vi "Timer_Restart.vi"(8 "Pass_Through_Time":dbl=-1.0 format="%33.4f", 11 "in Timer":T1 {"Accumulated TIme" format="%13.5p"; "StartTime" format="%13.5p"}) -> (3 "out Timer":T1 {"Accumulated TIme" format="%13.5p"; "StartTime" format="%13.5p"})   [LabVIEW 2019, in "Trajectory_Library.lvlib"]
doc: "Restart the timer by stopping the timer, if it is not already stopped, resetting the accumulated time, then starting the timer again. If you want an event to periodically reoccur at some time interval from the start time, consider using HasPeriodPassed instead.\n\nInputs:\n - Timer -- The Timer data cluster\n\nOutputs:\n - Timer -- The modified Timer data cluster"
uses:
  Trajectory_Library.lvlib
  TypeDef/TIMER.ctl
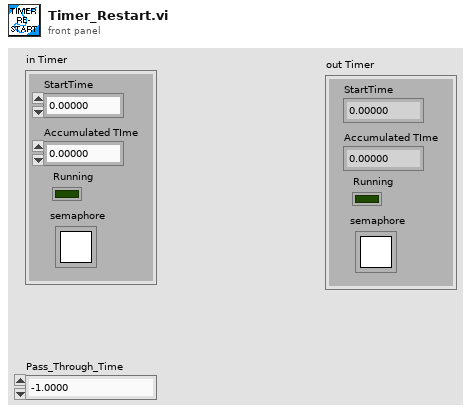
[diagram p1: front panel]
types:
  T1 = typedef "Trajectory_Library.lvlib/TIMER.ctl" = cluster{"StartTime":dbl, "Accumulated TIme":dbl, "Running":bool, "semaphore":T2}
  T2 = typedef "Semaphore RefNum" = refnum<k1>
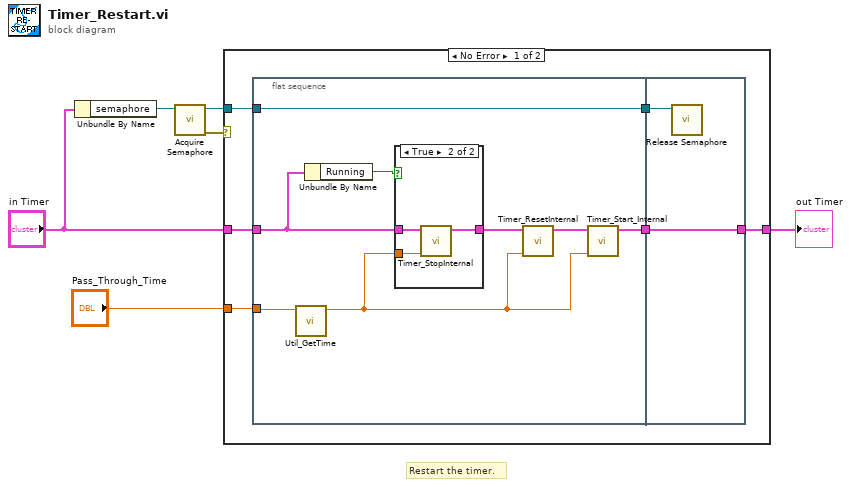
[diagram p0: block diagram]
diagram:
  # "Restart the timer."
  n1 = Unbundle By Name("in Timer") -> ("semaphore"=w4:T2)
  n2 = call <vilib>:"Acquire Semaphore.vi"("semaphore"=w4) -> ("error out"=w3:errorcluster, "semaphore out"=w2:T2)  [unwired: 4 in, 1 out]
  n3 = case shown="No Error" w3 {
    tunnel: "in Timer" -> [w12 w27]
    tunnel: [w11 w27] -> w6
    tunnel: w2 -> [w8 _]
    tunnel: "Pass_Through_Time" -> [w7 _]
    frame No Error {
      n4 = flat-sequence {
        tunnel: w12 -> [w17]
        tunnel: [w14] -> w10
        tunnel: [w20] -> w9
        tunnel: w8 -> [w20]
        tunnel: w7 -> [w16]
        tunnel: [w26] -> w11
        tunnel: w10 -> [w26]
        tunnel: w9 -> [w25]
        frame #0 {
          n5 = call "Util_GetTime.vi"("Pass_Through_Time"=w16) -> ("FPGA_Time_Seconds"=w13:dbl)  [unwired: 8 in, 2 out]
          n6 = Unbundle By Name(w17) -> ("Running"=w18:bool)
          n7 = case shown="True" w18 {
            tunnel: w13 -> [_ w24]
            tunnel: [w21 w23] -> w19
            tunnel: w17 -> [w21 w22]
            frame False {
            }
            frame True {
              n8 = call "Timer_StopInternal.vi"("Pass_Through_Time"=w24, "in Timer"=w22) -> ("out Timer"=w23:T1)  [unwired: 9 in]
            }
          }
          n9 = call "Timer_ResetInternal.vi"("Pass_Through_Time"=w13, "in TIMER"=w19) -> ("out TIMER"=w15:T1)  [unwired: 9 in]
          n10 = call "Timer_Start_Internal.vi"("FPGA_Time_Seconds"=w13, "in Timer in"=w15) -> ("in Timer out"=w14:T1)  [unwired: 9 in]
        }
        frame #1 {
          n11 = call <vilib>:"Release Semaphore.vi"("semaphore"=w25) -> ()  [unwired: 5 in, 2 out]
        }
      }
    }
    frame Error {
    }
  }
  "out Timer" <- w6
